vi "SQL_Destroy.vi"(8 "error in (no error)":errorcluster, 11 "reference in":refnum<class "SQL.lvclass">) -> (0 "error out":errorcluster, 3 "reference out":refnum<class "SQL.lvclass">)   [LabVIEW 2012, in "SQL.lvclass"]
uses:
  SQL.lvclass
  <vilib>/addons/database/NI_Database_API.lvlib
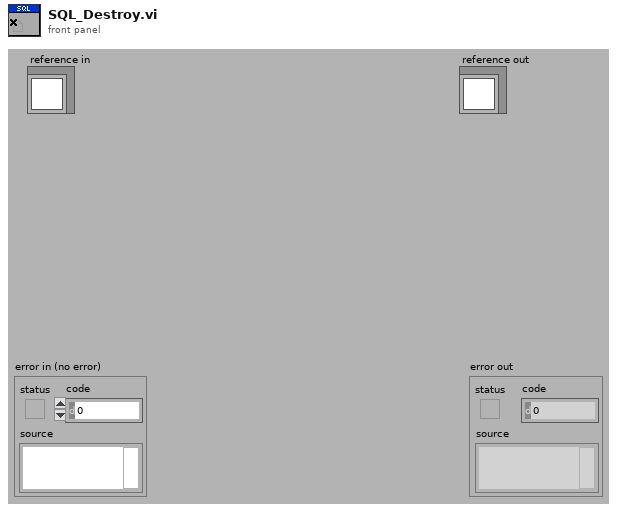
[diagram p1: front panel]
types:
  T1 = typedef "SQL.lvclass/ObjectAttributes.ctl" = cluster{"DB Connection Reference":T2}
  T2 = typedef "NI_Database_API.lvlib/Conn ObjectReference.ctl" = refnum<k1>
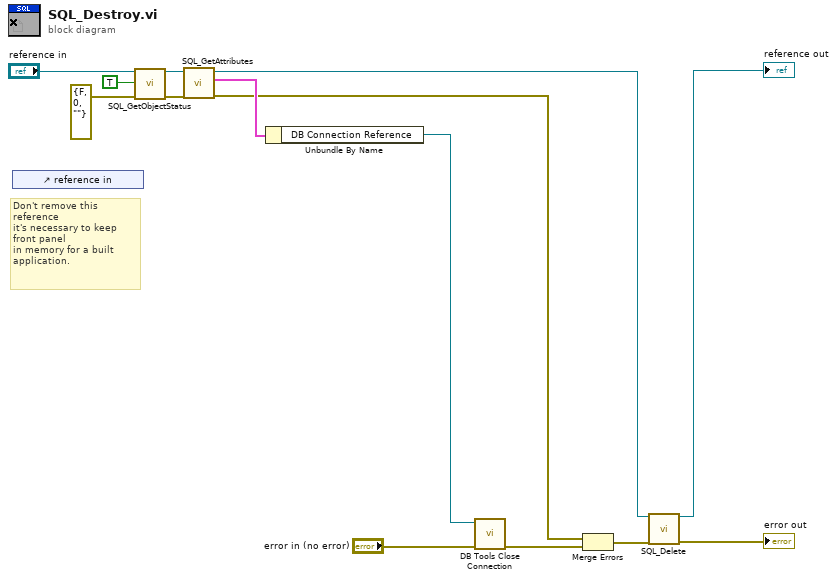
[diagram p0: block diagram]
diagram:
  # "Don't remove this reference\nit's necessary to keep front panel\nin memory for a built application."
  n1 = control-ref of="reference in"() -> ()  [unwired: 1 out]
  n2 = call "SQL_GetObjectStatus.vi"("reference in"="reference in", "Simple Info"=TRUE, "error in (no error)"=errorcluster {"status"=FALSE, "code"=0, "source"=""}) -> ("reference out"=w9:refnum<class "SQL.lvclass">, "error out"=w10:errorcluster)  [unwired: 3 in, 8 out]
  n3 = call "SQL_GetAttributes.vi"("error in (no error)"=w10, "reference in"=w9) -> ("error out"=w2:errorcluster, "Attributes"=w4:T1, "reference out"=w13:refnum<class "SQL.lvclass">)  [unwired: 6 in, 1 out]
  n4 = Unbundle By Name(w4) -> ("DB Connection Reference"=w3:T2)
  n5 = call <vilib>:"DB Tools Close Connection.vi"("error in (no error)"="error in (no error)", "connection reference"=w3) -> ("error out"=w1:errorcluster)  [unwired: 5 in]
  n6 = Merge Errors(w2, w1) -> (w12:errorcluster)
  n7 = call "SQL_Delete.vi"("reference in"=w13, "error in (no error)"=w12) -> ("reference out"=→"reference out":refnum<class "SQL.lvclass">, "error out"=→"error out":errorcluster)  [unwired: 15 in, 1 out]
